vi "4Pi 4Pi Modes - Deform Mirror DUAL AE V2.vi"(0 "DM Handles":T1(array[cluster]), 1 "Action":T2, 7 "Flats":dbl[](array[numeric]), 11 "Control Matrix":dbl[][](array[numeric])) -> (4 "DM Handles Out":T1(array[cluster]), 8 "Flats Out":dbl[](array[numeric]), 15 "Control Matrix Out":dbl[][](array[numeric]))   [LabVIEW 2016]
uses:
  4Pi 4Pi Modes - Controls/4Pi 4Pi Modes - Standard Action.ctl
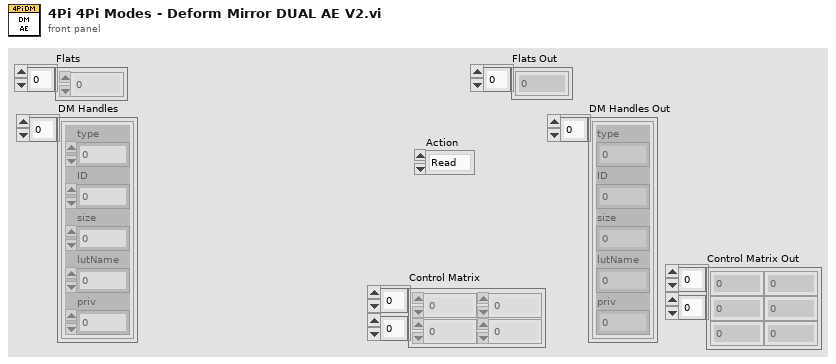
[diagram p1: front panel]
types:
  T1 = cluster{"type":i16, "ID":i16, "size":i32, "lutName":u64, "priv":u64}[]
  T2 = typedef "4Pi 4Pi Modes - Standard Action.ctl" = enum16{"Read", "Write"}
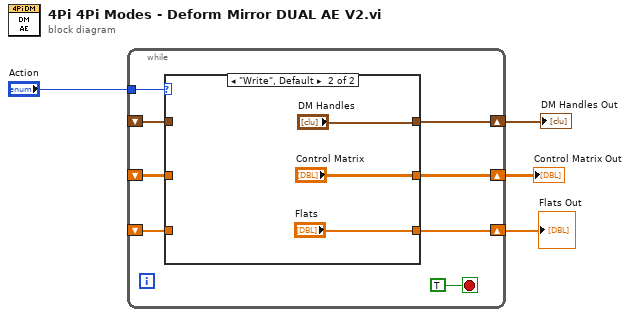
[diagram p0: block diagram]
diagram:
  n1 = while {
    tunnel: "Action" -> [w11]
    shift-right: [w7] -> w2
    shift-left: _ -> [w10]
    shift-right: [w9] -> w3
    shift-left: _ -> [w8]
    shift-right: [w6] -> w1
    shift-left: _ -> [w5]
    stop <- TRUE stop-if-true
    n2 = case shown="\"Write\", Default" w11 {
      tunnel: w10 -> [w14 _]
      tunnel: [w15 "Control Matrix"] -> w9
      tunnel: w8 -> [w15 _]
      tunnel: [w14 "Flats"] -> w7
      tunnel: [w13 "DM Handles"] -> w6
      tunnel: w5 -> [w13 _]
      frame "Read" {
      }
      frame "Write", Default {
      }
    }
  }
  "Control Matrix Out" <- w3
  "Flats Out" <- w2
  "DM Handles Out" <- w1
